vi "setTime.vi"(8 "error in (no error)":errorcluster, 11 "Time in":refnum<class "Time.lvclass">) -> (0 "error out":errorcluster, 3 "Time out":refnum<class "Time.lvclass">)   [LabVIEW 2015, in "Time.lvclass"]
uses:
  Time.lvclass
  Time.lvclass/Time.ctl
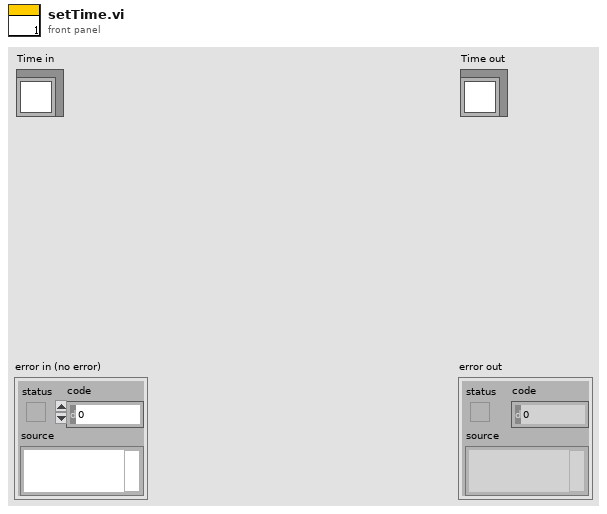
[diagram p1: front panel]
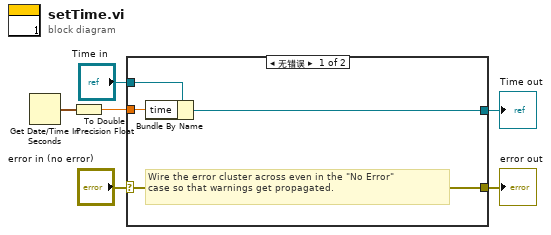
[diagram p0: block diagram]
diagram:
  n1 = Get Date/Time In Seconds() -> (seconds since 1Jan1904=w2:timestamp)
  n2 = To Double Precision Float(number=w2) -> (double precision float=w1:dbl)
  n3 = case shown="无错误" "error in (no error)" {
    selector: "error in (no error)" -> [w10 w12]
    tunnel: [w10 w12] -> w5
    tunnel: [w8 w11] -> w3
    tunnel: "Time in" -> [w9 w11]
    tunnel: w1 -> [w7 _]
    frame No Error {
      # "Wire the error cluster across even in the \"No Error\"\ncase so that warnings get propagated."
      n4 = Bundle By Name(cluster=w9, "time"=w7) -> (w8:refnum<class "Time.lvclass">)
    }
    frame Error {
    }
  }
  "error out" <- w5
  "Time out" <- w3
